vi "Part Number.vi"(8 "Value from LPCA":string, 10 "Command":T1(ring)) -> (0 "Prts Number":string, 1 "Part Number":string, 2 "Prts Index":i32, 3 "Part Index":i32, 4 "Prta Number":string, 5 "Prta Index":i32)   [LabVIEW 2017]
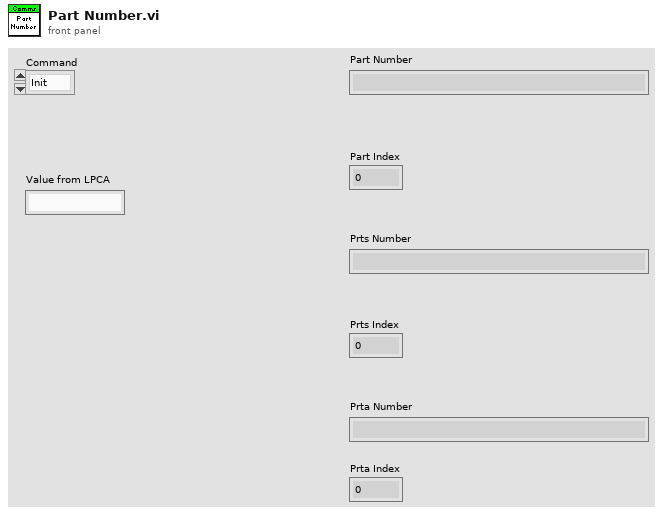
[diagram p1: front panel]
types:
  T1 = enum16{"Init", "Get Index", "Analyze Part", "Analyze Prts", "Analyze Prta", "Set VER", "Set TYPE"}
  T2 = cluster{"Part Hex Values":u8[], "Part Index":i32, "VER":string, "TYPE":string, "Prts Hex Values":u8[], "Prts Index":i32, "Prta Hex Values":u8[], "Prta Index":i32}
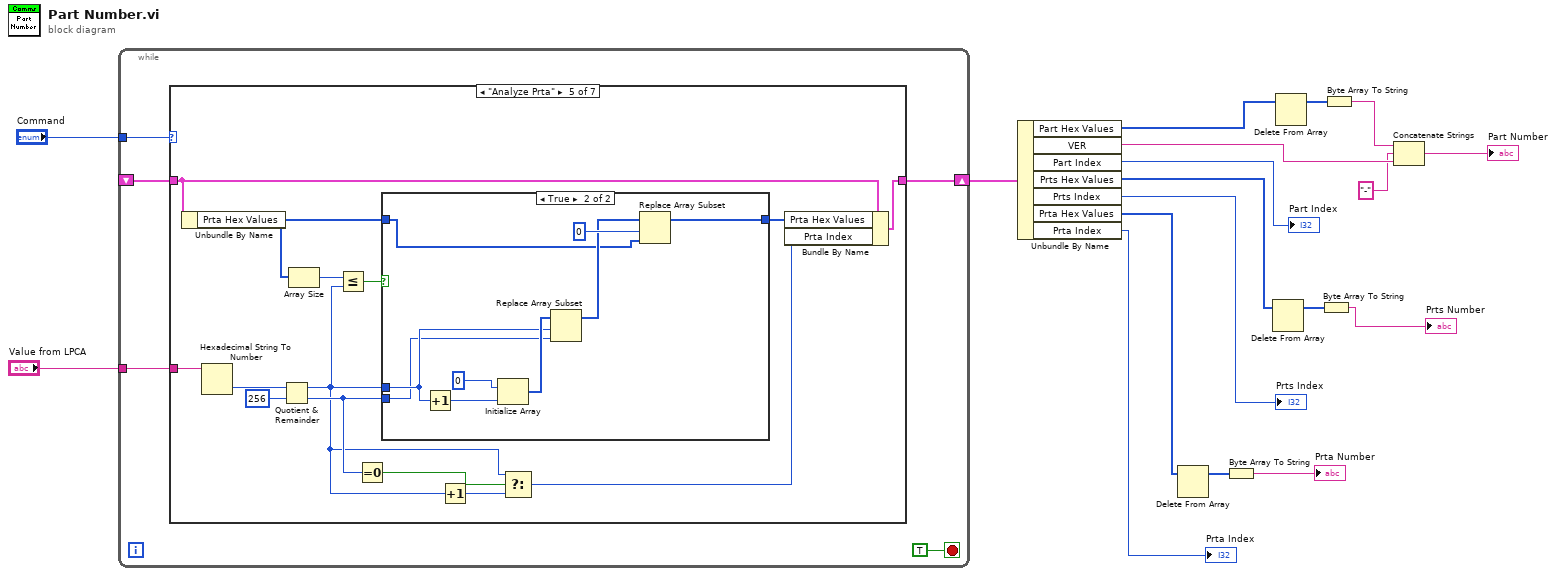
[diagram p0: block diagram]
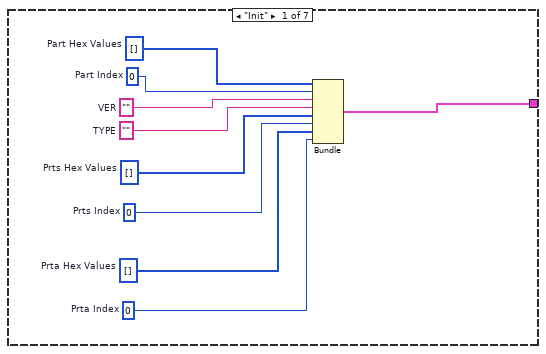
[diagram p2: hidden frame]
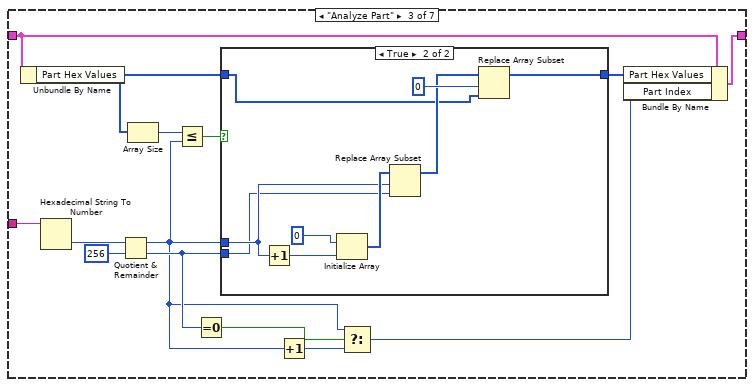
[diagram p4: hidden frame]
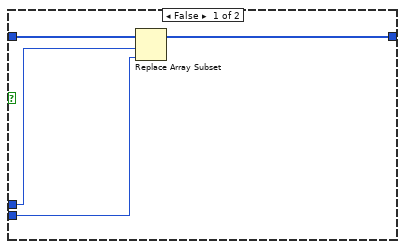
[diagram p5: hidden frame]
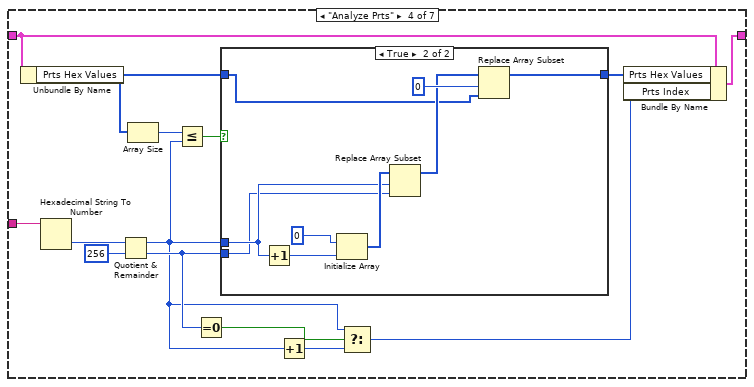
[diagram p6: hidden frame]
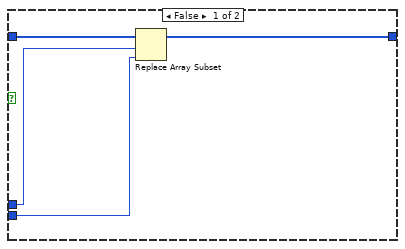
[diagram p7: hidden frame]
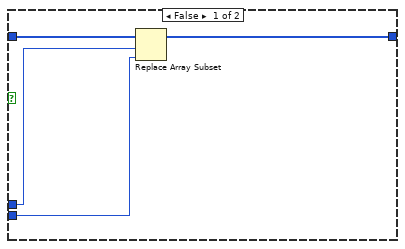
[diagram p8: hidden frame]
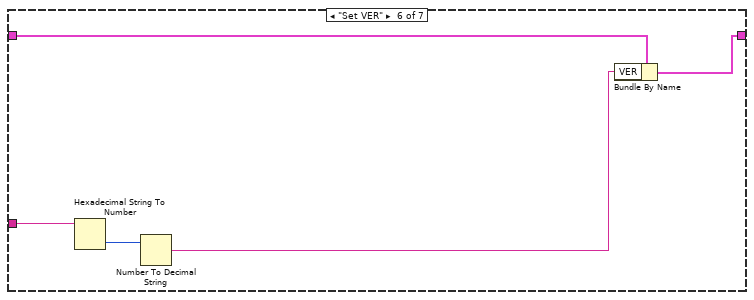
[diagram p9: hidden frame]
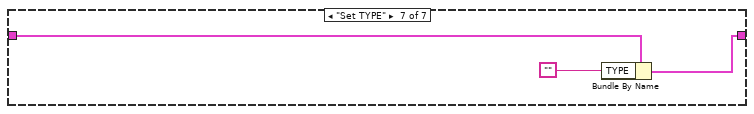
[diagram p10: hidden frame]
diagram:
  n1 = while {
    tunnel: "Command" -> [w23]
    tunnel: "Value from LPCA" -> [w22]
    shift-right: [w21] -> w16
    shift-left: _ -> [w20]
    stop <- TRUE stop-if-true
    n2 = case shown="\"Analyze Prta\"" w23 {
      tunnel: w22 -> [_ _ w46 w73 w100 w119 _]
      tunnel: [w30 w33 w47 w74 w101 w116 w121] -> w21
      tunnel: w20 -> [_ w33 w43 w70 w97 w117 w122]
      frame "Init" {
        w24 = 0  # Prta Index
        w25 = u8[] []  # Prta Hex Values
        w26 = 0  # Prts Index
        w27 = u8[] []  # Prts Hex Values
        w28 = ""  # TYPE
        w29 = ""  # VER
        w31 = 0  # Part Index
        w32 = u8[] []  # Part Hex Values
        n3 = Bundle("Part Hex Values"=w32, "Part Index"=w31, "VER"=w29, "TYPE"=w28, "Prts Hex Values"=w27, "Prts Index"=w26, "Prta Hex Values"=w25, "Prta Index"=w24) -> (w30:T2)  [unwired: 1 in]
      }
      frame "Get Index" {
      }
      frame "Analyze Part" {
        n4 = Unbundle By Name(w43) -> ("Part Hex Values"=w40:u8[])
        n5 = Hexadecimal String To Number(string=w46) -> (number=w45:u32)  [unwired: 2 in, 1 out]
        n6 = Quotient & Remainder(x=w45, y=u32 256) -> (x-y*floor(x/y)=w34:u32, floor(x/y)=w38:u32)
        n7 = Array Size(array=w40) -> (size(s)=w42:i32)
        n8 = Less Or Equal?(x=w42, y=w34) -> (x <= y?=w41:bool)
        n9 = Equal To 0?(x=w38) -> (x = 0?=w35:bool)
        n10 = case shown="True" w41 {
          tunnel: w40 -> [w51 w52]
          tunnel: w34 -> [w49 w57]
          tunnel: w38 -> [w50 w56]
          tunnel: [w48 w54] -> w39
          frame False {
            n11 = Replace Array Subset(array=w51, new element=w50, index=w49) -> (w48:u8[])
          }
          frame True {
            n12 = Increment(x=w57) -> (x+1=w59:u32)
            n13 = Initialize Array(u8 0, w59) -> (w58:u8[])
            n14 = Replace Array Subset(array=w58, new element=w56, index=w57) -> (w53:u8[])
            n15 = Replace Array Subset(array=w53, new element=w52, index=0) -> (w54:u8[])
          }
        }
        n16 = Increment(x=w34) -> (x+1=w37:u32)
        n17 = Select(t=w34, s=w35, f=w37) -> (s? t:f=w36:u32)
        n18 = Bundle By Name(cluster=w43, "Part Hex Values"=w39, "Part Index"=w36) -> (w47:T2)
      }
      frame "Analyze Prts" {
        n19 = Unbundle By Name(w70) -> ("Prts Hex Values"=w67:u8[])
        n20 = Hexadecimal String To Number(string=w73) -> (number=w72:u32)  [unwired: 2 in, 1 out]
        n21 = Quotient & Remainder(x=w72, y=u32 256) -> (x-y*floor(x/y)=w61:u32, floor(x/y)=w65:u32)
        n22 = Array Size(array=w67) -> (size(s)=w69:i32)
        n23 = Less Or Equal?(x=w69, y=w61) -> (x <= y?=w68:bool)
        n24 = Equal To 0?(x=w65) -> (x = 0?=w62:bool)
        n25 = case shown="True" w68 {
          tunnel: w67 -> [w78 w79]
          tunnel: w61 -> [w76 w84]
          tunnel: w65 -> [w77 w83]
          tunnel: [w75 w81] -> w66
          frame False {
            n26 = Replace Array Subset(array=w78, new element=w77, index=w76) -> (w75:u8[])
          }
          frame True {
            n27 = Increment(x=w84) -> (x+1=w86:u32)
            n28 = Initialize Array(u8 0, w86) -> (w85:u8[])
            n29 = Replace Array Subset(array=w85, new element=w83, index=w84) -> (w80:u8[])
            n30 = Replace Array Subset(array=w80, new element=w79, index=0) -> (w81:u8[])
          }
        }
        n31 = Increment(x=w61) -> (x+1=w64:u32)
        n32 = Select(t=w61, s=w62, f=w64) -> (s? t:f=w63:u32)
        n33 = Bundle By Name(cluster=w70, "Prts Hex Values"=w66, "Prts Index"=w63) -> (w74:T2)
      }
      frame "Analyze Prta" {
        n34 = Unbundle By Name(w97) -> ("Prta Hex Values"=w94:u8[])
        n35 = Hexadecimal String To Number(string=w100) -> (number=w99:u32)  [unwired: 2 in, 1 out]
        n36 = Quotient & Remainder(x=w99, y=u32 256) -> (x-y*floor(x/y)=w88:u32, floor(x/y)=w92:u32)
        n37 = Array Size(array=w94) -> (size(s)=w96:i32)
        n38 = Less Or Equal?(x=w96, y=w88) -> (x <= y?=w95:bool)
        n39 = Equal To 0?(x=w92) -> (x = 0?=w89:bool)
        n40 = case shown="True" w95 {
          tunnel: w94 -> [w105 w106]
          tunnel: w88 -> [w103 w111]
          tunnel: w92 -> [w104 w110]
          tunnel: [w102 w108] -> w93
          frame False {
            n41 = Replace Array Subset(array=w105, new element=w104, index=w103) -> (w102:u8[])
          }
          frame True {
            n42 = Increment(x=w111) -> (x+1=w113:u32)
            n43 = Initialize Array(u8 0, w113) -> (w112:u8[])
            n44 = Replace Array Subset(array=w112, new element=w110, index=w111) -> (w107:u8[])
            n45 = Replace Array Subset(array=w107, new element=w106, index=0) -> (w108:u8[])
          }
        }
        n46 = Increment(x=w88) -> (x+1=w91:u32)
        n47 = Select(t=w88, s=w89, f=w91) -> (s? t:f=w90:u32)
        n48 = Bundle By Name(cluster=w97, "Prta Hex Values"=w93, "Prta Index"=w90) -> (w101:T2)
      }
      frame "Set VER" {
        n49 = Hexadecimal String To Number(string=w119) -> (number=w118:u32)  [unwired: 2 in, 1 out]
        n50 = Number To Decimal String(number=w118) -> (decimal integer string=w115:string)  [unwired: 1 in]
        n51 = Bundle By Name(cluster=w117, "VER"=w115) -> (w116:T2)
      }
      frame "Set TYPE" {
        n52 = Bundle By Name(cluster=w122, "TYPE"="") -> (w121:T2)
      }
    }
  }
  n53 = Unbundle By Name(w16) -> ("Part Hex Values"=w10:u8[], "VER"=w14:string, "Part Index"=→"Part Index":i32, "Prts Hex Values"=w7:u8[], "Prts Index"=→"Prts Index":i32, "Prta Hex Values"=w1:u8[], "Prta Index"=→"Prta Index":i32)
  n54 = Delete From Array(array=w1) -> (array with subset deleted=w3:u8[])  [unwired: 2 in, 1 out]
  n55 = Byte Array To String(unsigned byte array=w3) -> (string=→"Prta Number":string)
  n56 = Delete From Array(array=w7) -> (array with subset deleted=w8:u8[])  [unwired: 2 in, 1 out]
  n57 = Delete From Array(array=w10) -> (array with subset deleted=w9:u8[])  [unwired: 2 in, 1 out]
  n58 = Byte Array To String(unsigned byte array=w8) -> (string=→"Prts Number":string)
  n59 = Byte Array To String(unsigned byte array=w9) -> (string=w13:string)
  n60 = Concatenate Strings(w13, "-", w14) -> (→"Part Number":string)
